vi "getSettingPageNames.vi"(11 "Setting in":refnum<class "Setting.lvclass">) -> (2 "SettingPageNames":string[](array[string]), 3 "Setting out":refnum<class "Setting.lvclass">)   [LabVIEW 2016, in "Setting.lvclass"]
uses:
  Setting.lvclass
  Setting.lvclass/Setting.ctl
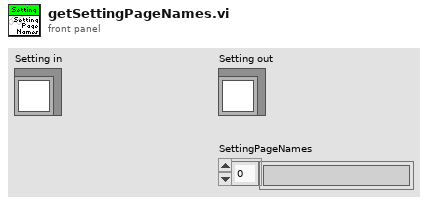
[diagram p1: front panel]
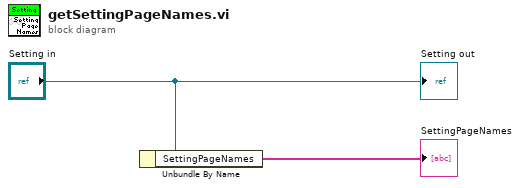
[diagram p0: block diagram]
diagram:
  n1 = Unbundle By Name("Setting in") -> ("SettingPageNames"=→"SettingPageNames":string[])
  "Setting out" <- "Setting in"
